vi "Close Interlock.vi"(8 "error in (no error)":errorcluster, 11 "Interlock Sample in":refnum<class "Interlock Sample.lvclass">) -> (0 "error out":errorcluster, 3 "Interlock Sample out":refnum<class "Interlock Sample.lvclass">)   [LabVIEW 2015, in "cRIO-Carbondioxide.lvlib" / "Interlock Sample.lvclass"]
uses:
  Interlock Sample.lvclass
  Interlock/Interlock.lvclass
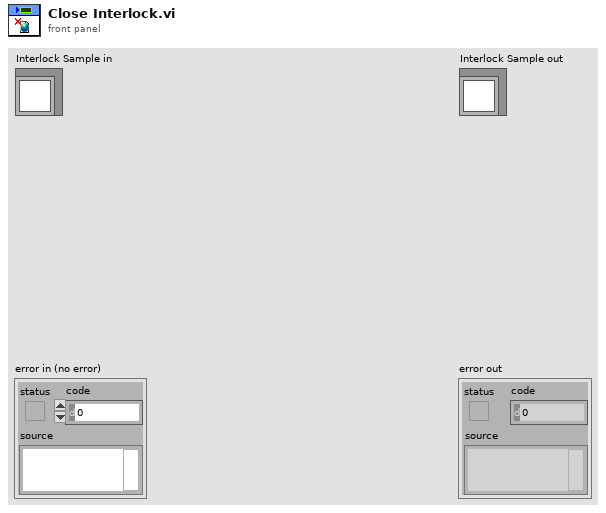
[diagram p1: front panel]
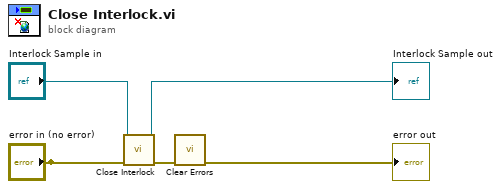
[diagram p0: block diagram]
diagram:
  n1 = call-parent "Close Interlock.vi"("error in (no error)"="error in (no error)", "Interlock in"="Interlock Sample in") -> ("error out"=w2:errorcluster, "Interlock out"=→"Interlock Sample out":refnum<class "Interlock Sample.lvclass">)  [unwired: 8 in]
  n2 = call <vilib>:"Clear Errors.vi"("error in (no error)"=w2) -> ()  [unwired: 5 in, 2 out]
  "error out" <- "error in (no error)"
